vi "Gradient Read Single.vi"(8 "error in":errorcluster, 9 "Channel Index":i32=1, 11 "Voltage Gradient in":refnum<class "Voltage Gradient.lvclass">) -> (0 "error out":errorcluster, 1 "Changed or First Call?":bool, 2 "Voltage SP":dbl, 3 "Voltage Gradient out":refnum<class "Voltage Gradient.lvclass">)   [LabVIEW 2023, in "Voltage Gradient.lvclass"]
uses:
  Voltage Gradient.lvclass
  Voltage Gradient.lvclass/Voltage Gradient.ctl
  Parents/Gradient/Gradient.lvclass
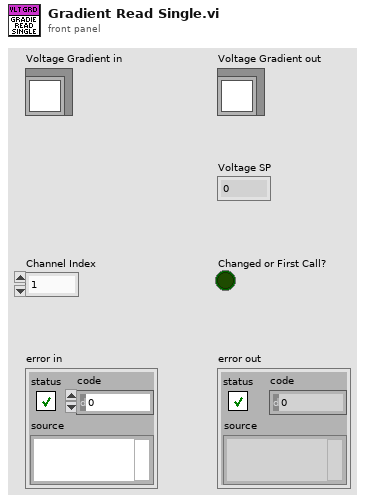
[diagram p1: front panel]
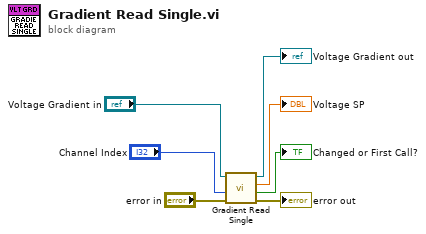
[diagram p0: block diagram]
diagram:
  n1 = call-parent "Gradient Read Single.vi"("error in"="error in", "Channel Index"="Channel Index", "Gradient in"="Voltage Gradient in") -> ("error out"=→"error out":errorcluster, "Changed or First Call?"=→"Changed or First Call?":bool, "Current SP"=→"Voltage SP":dbl, "Gradient out"=→"Voltage Gradient out":refnum<class "Voltage Gradient.lvclass">)  [unwired: 5 in]
